vi "electrodes.vi"(4 "electrodes/ cell":i32=5, 6 "cell length (m)":dbl=0.02 format="%#_6p", 7 "phase / 2 pi":dbl, 9 "velocity":dbl[](array[numeric]), 10 "position":dbl[](array[numeric]), 11 "time":dbl[](array[numeric])) -> (2 "frequency":dbl[](array[numeric]), 3 "waveforms":dbl[][](array[numeric]))   [LabVIEW 2013, in "wf_tools.lvlib"]
uses:
  wf_tools.lvlib
panel:
  out "frequency t":cluster{"time":dbl[], dbl[]}(graph)
  out "frequency x":cluster{"position":dbl[], dbl[]}(graph)
  out "waveform x":cluster{"time":dbl[], dbl[]}[](graph)
  out "waveform t":cluster{"time":dbl[], dbl[]}[](graph)
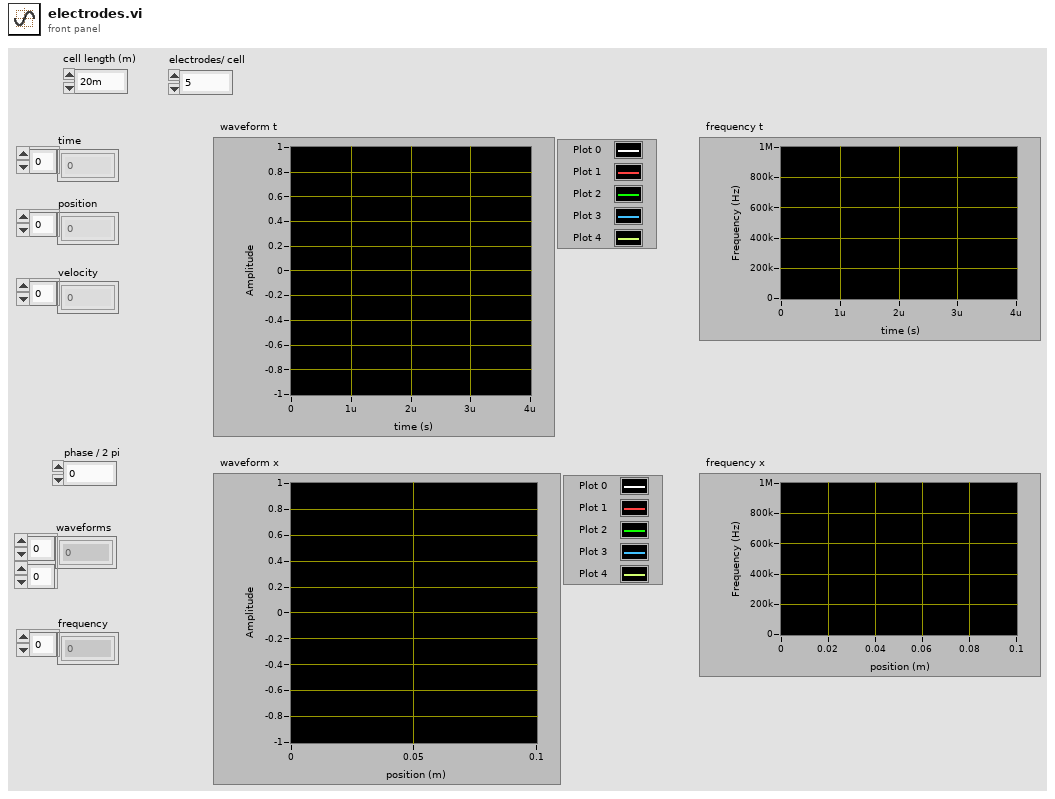
[diagram p1: front panel]
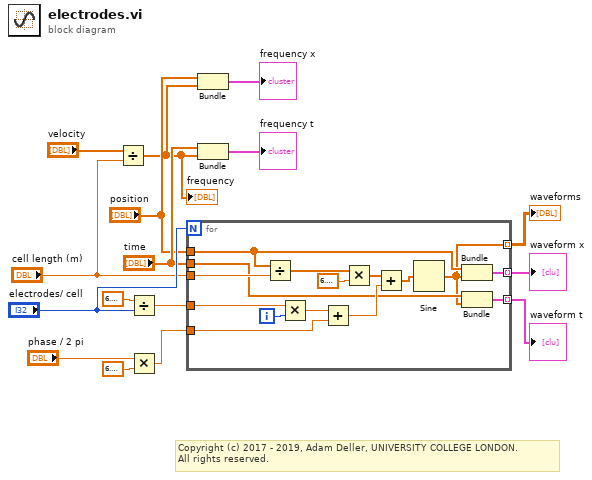
[diagram p0: block diagram]
diagram:
  # "Copyright (c) 2017 - 2019, Adam Deller, UNIVERSITY COLLEGE LONDON.\nAll rights reserved."
  n1 = Divide(x="velocity", y="cell length (m)") -> (x/y=w3:dbl[])
  "frequency" <- w3
  n2 = Divide(x=6.283185307179586, y="electrodes/ cell") -> (x/y=w14:dbl)
  n3 = Multiply(x="phase / 2 pi", y=6.283185307179586) -> (x*y=w6:dbl)
  n4 = for {
    N: "electrodes/ cell" -> [_]
    tunnel: w14 -> [w30]
    tunnel: "time" -> [w19]
    tunnel: "position" -> [w18]
    tunnel: "cell length (m)" -> [w20]
    tunnel: [w29] -> w9 mode=indexing
    tunnel: [w24] -> w10 mode=indexing
    tunnel: w6 -> [w22]
    tunnel: [w17] -> w5 mode=indexing
    i -> [w31]
    n5 = Divide(x=w18, y=w20) -> (x/y=w27:dbl[])
    n6 = Multiply(x=w30, y=w31) -> (x*y=w23:dbl)
    n7 = Add(x=w23, y=w22) -> (x+y=w21:dbl)
    n8 = Multiply(x=w27, y=6.283185307179586) -> (x*y=w25:dbl[])
    n9 = Add(x=w25, y=w21) -> (x+y=w28:dbl[])
    n10 = Sine(x=w28) -> (sin(x)=w17:dbl[])
    n11 = Bundle("position"=w18, w17) -> (w24:cluster{"position":dbl[], dbl[]})  [unwired: 1 in]
    n12 = Bundle("time"=w19, w17) -> (w29:cluster{"time":dbl[], dbl[]})  [unwired: 1 in]
  }
  "waveform t" <- w9
  "waveform x" <- w10
  "waveforms" <- w5
  n13 = Bundle("position"="position", w3) -> (→"frequency x":cluster{"position":dbl[], dbl[]})  [unwired: 1 in]
  n14 = Bundle("time"="time", w3) -> (→"frequency t":cluster{"time":dbl[], dbl[]})  [unwired: 1 in]
